vi "LoadWorldWithFood.vi"(1 "Input Array":i8[][](array[numeric]), 2 "Food per Level":i32) -> (0 "Output Array":i8[][](array[numeric]))   [LabVIEW 2014]
doc: "Loads a 10x10 occupancy grid with N food squares valued 1 to N."
panel:
  # "This VI places N food squares into the world, with one of each of the valuews from 1 to N:"
  # "food per level"
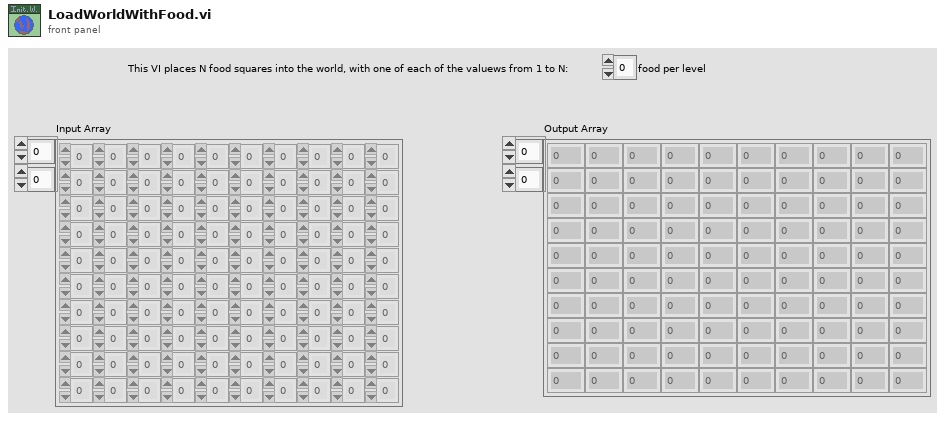
[diagram p1: front panel]
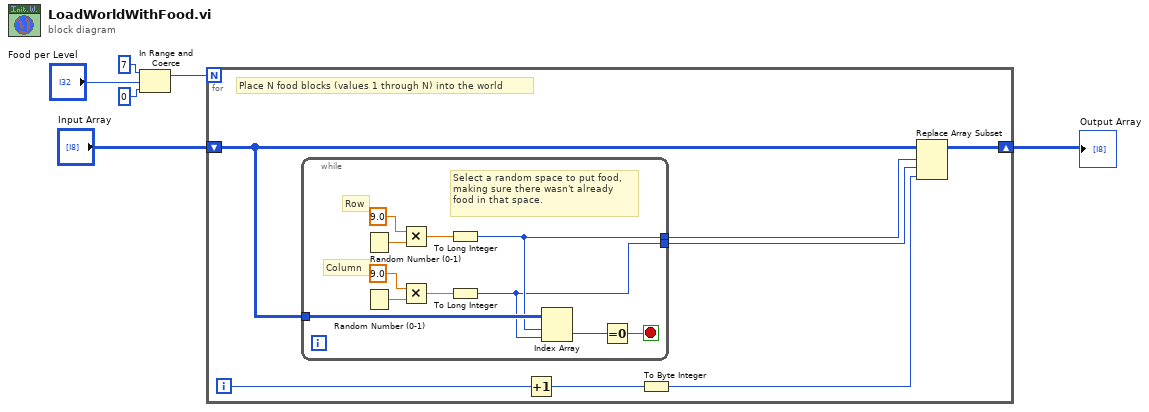
[diagram p0: block diagram]
diagram:
  n1 = In Range and Coerce(upper limit=7, x="Food per Level", lower limit=0) -> (coerced(x)=w2:i32)  [unwired: 1 out]
  n2 = for {
    N: w2 -> [_]
    shift-right: [w13] -> w1
    shift-left: "Input Array" -> [w12]
    i -> [w9]
    # "Place N food blocks (values 1 through N) into the world"
    n3 = while {
      tunnel: w12 -> [w24]
      tunnel: [w15] -> w11
      tunnel: [w14] -> w10
      stop <- w16 stop-if-true
      # "Select a random space to put food,\nmaking sure there wasn't already \nfood in that space."
      # "Column"
      # "Row"
      n4 = Random Number (0-1)() -> (number: 0 to 1=w23:dbl)
      n5 = Random Number (0-1)() -> (number: 0 to 1=w20:dbl)
      n6 = Multiply(x=9.0 ("y"), y=w23) -> (x*y=w19:dbl)
      n7 = Multiply(x=9.0 ("y"), y=w20) -> (x*y=w18:dbl)
      n8 = To Long Integer(number=w19) -> (32bit integer=w15:i32)
      n9 = To Long Integer(number=w18) -> (32bit integer=w14:i32)
      n10 = Index Array(array=w24, index (row)=w15, index (col)=w14) -> (element=w17:i8)
      n11 = Equal To 0?(x=w17) -> (x = 0?=w16:bool)
    }
    n12 = Increment(x=w9) -> (x+1=w8:i32)
    n13 = To Byte Integer(number=w8) -> (8bit integer=w7:i8)
    n14 = Replace Array Subset(array=w12, new element=w7, index (row)=w11, index (col)=w10) -> (w13:i8[][])
  }
  "Output Array" <- w1
